vi "Get Console_Q.vi"(8 "error in (no error)":errorcluster, 11 "Console Reply.lvclass":refnum<class "Console Reply.lvclass">) -> (0 "error out":errorcluster, 2 "Console Q":refnum<class "Message Enqueuer.lvclass">, 3 "Console Reply.lvclass":refnum<class "Console Reply.lvclass">)   [LabVIEW 2015, in "EditPanel API.lvlib" / "Console Reply.lvclass"]
uses:
  Console Reply.lvclass
  <vilib>/ActorFramework/Message Enqueuer/Message Enqueuer.lvclass
  Console Reply.lvclass/Console Reply.ctl
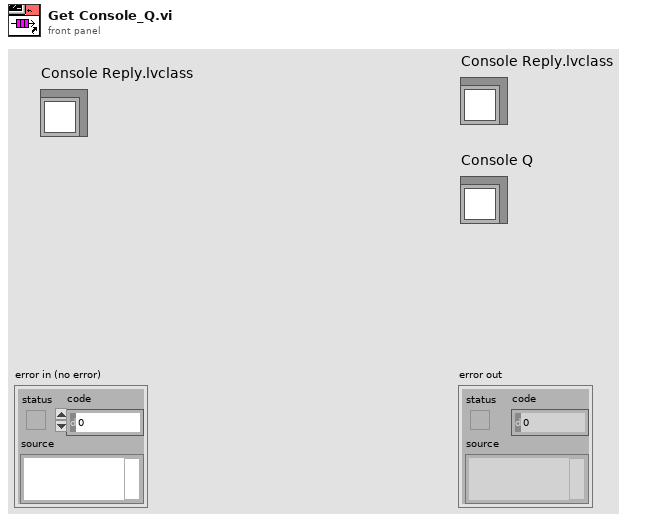
[diagram p1: front panel]
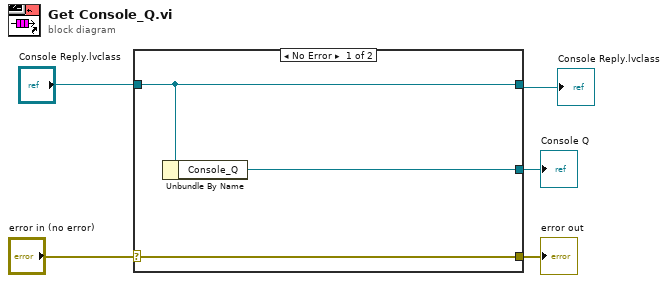
[diagram p0: block diagram]
diagram:
  n1 = case shown="No Error" "error in (no error)" {
    selector: "error in (no error)" -> [w8 w9]
    tunnel: [w8 w9] -> w4
    tunnel: [w7 w10] -> w1
    tunnel: "Console Reply.lvclass" -> [w7 w10]
    tunnel: [w6 _] -> w3
    frame No Error {
      n2 = Unbundle By Name(w7) -> ("Console_Q"=w6:refnum<class "Message Enqueuer.lvclass">)
    }
    frame Error {
    }
  }
  "error out" <- w4
  "Console Q" <- w3
  "Console Reply.lvclass" <- w1
